vi "ADC_Bulk_Wrapper.vi"(4 "oversamples":u8, 5 "Process Data?":bool, 6 "# channels":u8, 7 "DeviceIndex":u32, 8 "error in (no error)":errorcluster, 9 "Gains In":T1[](array[typedef]), 10 "Action":T2, 11 "BufSize(32bit samples)":u32) -> (0 "error out":errorcluster, 1 "pBuf":u16[](graph), 2 "Data":dbl[][](array[numeric]), 3 "Actual BufSize":u32)   [LabVIEW 8.6]
doc: "Calls the ADC Bulk Read functionality\n\nCall this first with Action set to: Start Read\nDeviceIndex, BufSize, Gains, # Channs, and Oversamples must be specified in Start Read mode only.\n\n\nThen, periodically call with Action set to: Read Buffer to retrieve data thus far."
uses:
  Windows/System32/AIOUSB.dll
  <vilib>/Analysis/NI_AALBase.lvlib
  Controls/Bulk Wrapper Action.ctl
  Controls/Gain Mode.ctl
panel:
  out "Elapsed Time (ms)":u32
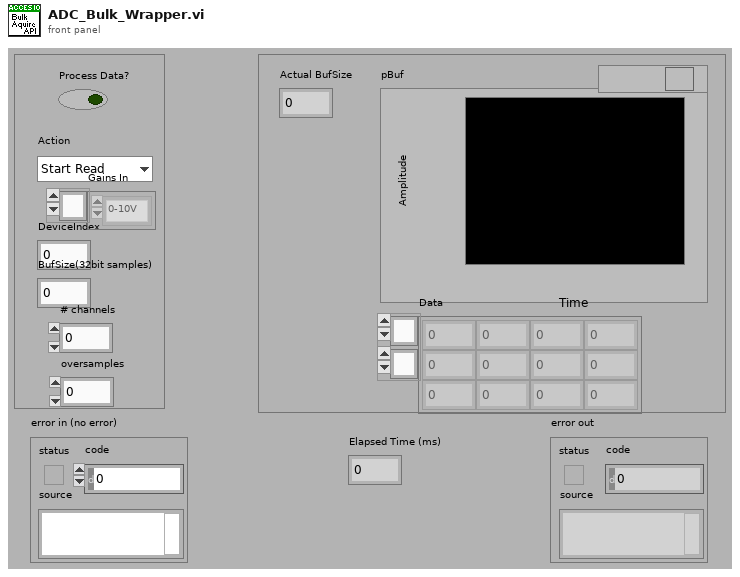
[diagram p1: front panel]
types:
  T1 = typedef "Gain Mode.ctl" = enum8{"0-10V", "+/- 10V", "0-5V", "+/- 5V", "0-2V", "+/- 2V", "0-1V", "+/- 1V"}
  T2 = typedef "Bulk Wrapper Action.ctl" = enum16{"Start Read", "Read Buffer"}
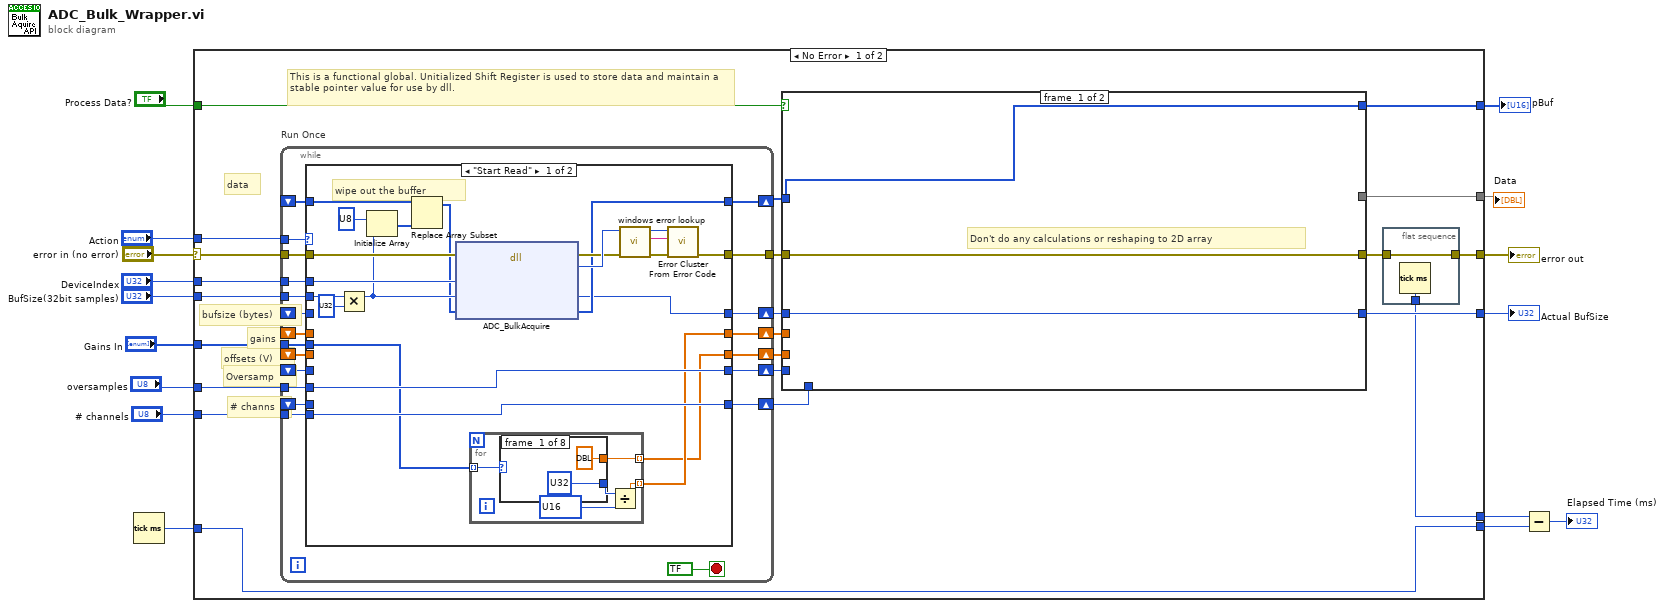
[diagram p0: block diagram]
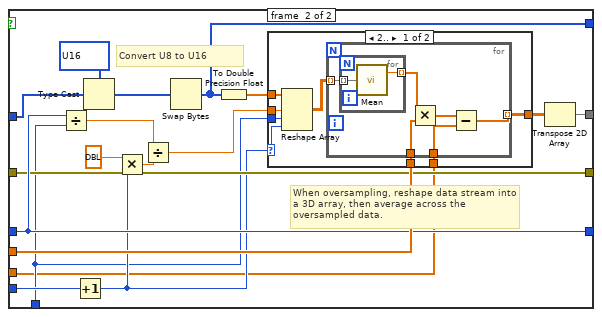
[diagram p2: hidden frame]
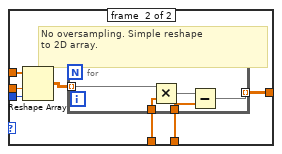
[diagram p3: hidden frame]
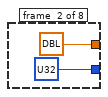
[diagram p4: hidden frame]
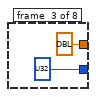
[diagram p5: hidden frame]
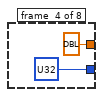
[diagram p6: hidden frame]
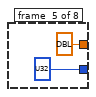
[diagram p7: hidden frame]
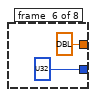
[diagram p8: hidden frame]
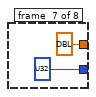
[diagram p9: hidden frame]
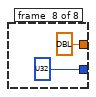
[diagram p10: hidden frame]
diagram:
  n1 = Tick Count (ms)() -> (millisecond timer value=w4:u32)
  n2 = case shown="No Error" "error in (no error)" {
    selector: "error in (no error)" -> [w34 w160]
    tunnel: [w22 w160] -> w16
    tunnel: "Action" -> [w37 _]
    tunnel: "DeviceIndex" -> [w36 _]
    tunnel: "BufSize(32bit samples)" -> [w35 _]
    tunnel: [w23 _] -> w11
    tunnel: "Gains In" -> [w33 _]
    tunnel: "oversamples" -> [w32 _]
    tunnel: "# channels" -> [w31 _]
    tunnel: [w26 _] -> w7
    tunnel: [w27 _] -> w6
    tunnel: "Process Data?" -> [w25 _]
    tunnel: w4 -> [w19 _]
    tunnel: [w20 _] -> w3
    tunnel: [w19 _] -> w2
    frame #0 {
      # "offsets (V)"
      # "# channs"
      # "Oversamp"
      # "gains"
      # "bufsize (bytes)"
      # "data"
      # "This is a functional global. Unitialized Shift Register is used to store data and maintain a stable pointer value for use by dll."
      n3 = while "Run Once" {
        tunnel: w36 -> [w110]
        tunnel: [w109] -> w24
        tunnel: w34 -> [w103]
        tunnel: w35 -> [w107]
        shift-right: [w106] -> w38
        shift-left: _ -> [w104]
        tunnel: w37 -> [w105]
        shift-right: [w102] -> w30
        shift-left: _ -> [w101]
        shift-right: [w100] -> w28
        shift-left: _ -> [w96]
        shift-right: [w98] -> w18
        shift-left: _ -> [w95]
        tunnel: w33 -> [w99]
        tunnel: w32 -> [w97]
        shift-right: [w94] -> w29
        shift-left: _ -> [w92]
        tunnel: w31 -> [w93]
        shift-right: [w90] -> w17
        shift-left: _ -> [w91]
        stop <- bool ? stop-if-true
        n4 = case shown="\"Start Read\"" w105 {
          tunnel: w110 -> [w125 _]
          tunnel: [w131 w158] -> w109
          tunnel: w107 -> [w123 _]
          tunnel: [w122 w159] -> w106
          tunnel: w104 -> [w116 w159]
          tunnel: w103 -> [w126 w158]
          tunnel: [w121 w157] -> w102
          tunnel: w101 -> [_ w157]
          tunnel: [w117 w156] -> w100
          tunnel: w99 -> [w118 _]
          tunnel: [w120 w155] -> w98
          tunnel: w97 -> [w120 _]
          tunnel: w96 -> [_ w156]
          tunnel: w95 -> [_ w155]
          tunnel: [w119 w154] -> w94
          tunnel: w93 -> [w119 _]
          tunnel: w92 -> [_ w154]
          tunnel: w91 -> [_ w153]
          tunnel: [w111 w153] -> w90
          frame #0 {
            # "wipe out the buffer"
            n5 = Multiply(x=w123, y=u32 ?) -> (x*y=w114:u32)
            n6 = Initialize Array(u8 ? ("x"), w114) -> (w113:u8[])
            n7 = Replace Array Subset(array=w116, new element=w113) -> (w112:u8[])  [unwired: 1 in]
            n8 = dll-call lib="C:/Windows/System32/AIOUSB.dll" fn="ADC_BulkAcquire"(error in=w126, "DeviceIndex"=w125, "BufSize"=w114, "pBuf"=w112) -> (error out=w127:errorcluster, "return type"=w128:u32, "BufSize"=w121:u32, "pBuf"=w122:u8[])  [unwired: 3 in, 1 out]
            n9 = for {
              tunnel: w118 -> [w136] mode=indexing
              tunnel: [w133] -> w117 mode=indexing
              tunnel: [w132] -> w111 mode=indexing
              n10 = case shown="\"0-5V\"" w136 {
                tunnel: [u32 ? ("x") u32 ? ("x") u32 ? ("x") u32 ? ("x") u32 ? ("x") u32 ? ("x") u32 ? ("x") u32 ? ("x")] -> w134
                tunnel: [dbl ? dbl ? dbl ? dbl ? dbl ? dbl ? dbl ? dbl ?] -> w132
                frame #0 {
                }
                frame #1 {
                }
                frame #2 {
                }
                frame #3 {
                }
                frame #4 {
                }
                frame #5 {
                }
                frame #6 {
                }
                frame #7 {
                }
              }
              n11 = Divide(x=w134, y=u16 ? ("BlockIndex")) -> (x/y=w133:dbl)
            }
            n12 = call "windows error lookup.vi"("error in (no error)"=w127, "Error Code"=w128) -> ("error out"=w130:errorcluster, "error message (\"\")"=w129:string)  [unwired: 8 in]
            n13 = call <vilib>:"Error Cluster From Error Code.vi"("error in (no error)"=w130, "error message (\"\")"=w129, "error code (0)"=w128) -> ("error out"=w131:errorcluster)  [unwired: 6 in]
          }
          frame #1 {
          }
        }
      }
      n14 = case shown="True" w25 {
        tunnel: w38 -> [w42 w48]
        tunnel: w30 -> [w41 w55]
        tunnel: w29 -> [_ w45]
        tunnel: w28 -> [_ w58]
        tunnel: [w42 w47] -> w27
        tunnel: [_ w56] -> w26
        tunnel: [w43 w54] -> w21
        tunnel: w24 -> [w43 w54]
        tunnel: [w41 w55] -> w23
        tunnel: w18 -> [_ w53]
        tunnel: w17 -> [_ w44]
        frame #0 {
          # "Don't do any calculations or reshaping to 2D array"
        }
        frame #1 {
          # "When oversampling, reshape data stream into a 3D array, then average across the oversampled data."
          # "Convert U8 to U16"
          n15 = Divide(x=w55, y=w45) -> (x/y=w60:dbl)
          n16 = Increment(x=w53) -> (x+1=w49:u8)
          n17 = Type Cast(type=u16[] ? ("pBuf"), x=w48) -> (*(type *) &x=w46:u16[])
          n18 = Multiply(x=dbl ? ("y"), y=w49) -> (x*y=w50:dbl)
          n19 = Divide(x=w60, y=w50) -> (x/y=w59:dbl)
          n20 = Swap Bytes(anything=w46) -> (byte swapped=w47:u16[])
          n21 = To Double Precision Float(number=w47) -> (double precision float=w52:dbl[])
          n22 = case shown="2.." w49 {
            selector: w49 -> [w63 _]
            tunnel: w59 -> [w69 w84]
            tunnel: w45 -> [w68 w83]
            tunnel: w58 -> [w66 w81]
            tunnel: [w65 w80] -> w57
            tunnel: w52 -> [w64 w79]
            tunnel: w44 -> [w62 w78]
            frame #0 {
              n23 = Reshape Array(w64, w69, w68, w63) -> (w67:dbl[][][])
              n24 = for {
                tunnel: w67 -> [w75] mode=indexing
                tunnel: w66 -> [w73]
                tunnel: [w71] -> w65 mode=indexing
                tunnel: w62 -> [w70]
                n25 = for {
                  tunnel: w75 -> [w77] mode=indexing
                  tunnel: [w76] -> w74 mode=indexing
                  n26 = call <vilib>:"Mean.vi"("X"=w77) -> ("mean"=w76:dbl)  [unwired: 1 out]
                }
                n27 = Multiply(x=w74, y=w73) -> (x*y=w72:dbl[])
                n28 = Subtract(x=w72, y=w70) -> (x-y=w71:dbl[])
              }
            }
            frame #1 {
              # "No oversampling. Simple reshape\nto 2D array."
              n29 = Reshape Array(w79, w84, w83) -> (w82:dbl[][])
              n30 = for {
                tunnel: w82 -> [w87] mode=indexing
                tunnel: w81 -> [w89]
                tunnel: [w86] -> w80 mode=indexing
                tunnel: w78 -> [w85]
                n31 = Multiply(x=w87, y=w89) -> (x*y=w88:dbl[])
                n32 = Subtract(x=w88, y=w85) -> (x-y=w86:dbl[])
              }
            }
          }
          n33 = Transpose 2D Array(2D array=w57) -> (transposed array=w56:dbl[][])
        }
      }
      n34 = flat-sequence {
        tunnel: [w40] -> w22
        tunnel: w21 -> [w40]
        tunnel: [w39] -> w20
        frame #0 {
          n35 = Tick Count (ms)() -> (millisecond timer value=w39:u32)
        }
      }
    }
    frame #1 {
    }
  }
  "error out" <- w16
  "Actual BufSize" <- w11
  "pBuf" <- w6
  "Data" <- w7
  n36 = Subtract(x=w3, y=w2) -> (x-y=→"Elapsed Time (ms)":u32)
